vi "Scaling Params.vi"(8 "error in (no error)":errorcluster, 11 "Scaling in":refnum<class "Scaling Config.lvclass">) -> (0 "error out":errorcluster, 1 "Scale Params":dbl[][](array[numeric]), 2 "Scale Types":T1[](array[typedef]), 3 "Scaling out":refnum<class "Scaling Config.lvclass">)   [LabVIEW 2020, in "VolatusConfig.lvlib" / "Scaling Config.lvclass"]
uses:
  Scaling Config.lvclass
  C:/dev/lv20CE/relink/lv-volatus/VolatusConfig/VolatusConfigElement/VolatusConfigElement.lvclass
  Scale Type.ctl
  Meta Type.ctl
  SensorList/SensorList.lvclass
  Scaling Config.lvclass/Scaling Config.ctl
  VolatusConfigElement/VolatusConfigElement.lvclass/VolatusConfigElement.ctl
  VolatusConfigElement/Element.vi
  lv-cdm/CDM-Config/Config Lookup/Match Meta.vi
  lv-cdm/CDM-Config/Config Element/Owner.vi
  lv-cdm/CDM-Config/Config Manager/Lookup Descendant.vi
  lv-cdm/CDM-Config/Config Filter/Config Lookup.lvclass
  VolatusConfigElement/VolatusConfigElement.lvclass
  VolatusConfig.lvlib
  lv-cdm/CDM-Config/Config Element/Config Element.lvclass
  Scale/Scale Config.lvclass
  VolatusErrorUtilities/MultiErrors/MultiErrors.lvclass
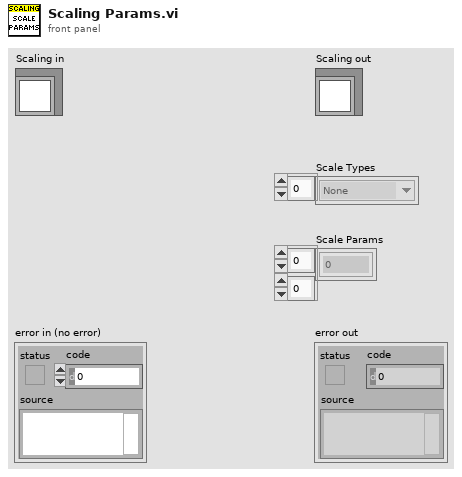
[diagram p1: front panel]
types:
  T1 = typedef "VolatusConfig.lvlib/Scale Type.ctl" = enum16{"None", "Sensor", "Polynomial", "Threshold", "Invert Bool", "Exponential"}
  T2 = typedef "VolatusConfig.lvlib/Meta Type.ctl" = enum16{"UNKNOWN", "VL_System", "VL_Cluster", "VL_Node", "VL_Task", "VL_Group", "VL_Channel", "VL_Task_List", "VL_Scaling", "VL_Sensor", "VL_Sensor_List", "VL_Scale"}
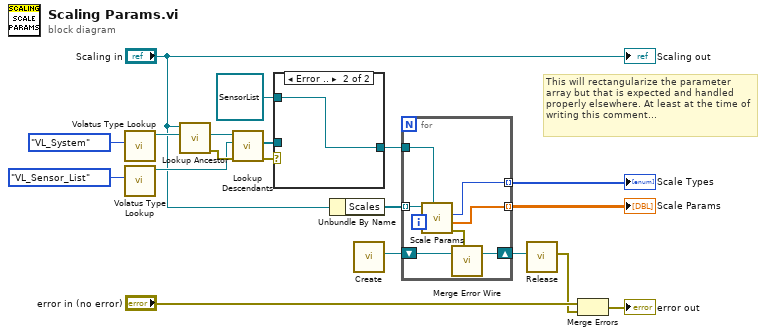
[diagram p0: block diagram]
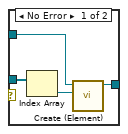
[diagram p2: hidden frame]
diagram:
  # "This will rectangularize the parameter array but that is expected and handled properly elsewhere. At least at the time of writing this comment..."
  n1 = call "Volatus Type Lookup.vi"("Meta Type"=Meta_Type."VL_System") -> ("Config Lookup out"=w18:refnum<class "Config Lookup.lvclass">)  [unwired: 9 in, 1 out]
  n2 = call "Volatus Type Lookup.vi"("Meta Type"=Meta_Type."VL_Sensor_List") -> ("Config Lookup out"=w14:refnum<class "Config Lookup.lvclass">)  [unwired: 9 in, 1 out]
  n3 = call "Lookup Ancestor.vi"("Lookup"=w18, "VolatusConfigElement in"="Scaling in") -> ("error out"=w19:errorcluster, "Ancestor"=w15:refnum<class "Config Element.lvclass">)  [unwired: 7 in, 1 out]
  n4 = call "Lookup Descendants.vi"("error in (no error)"=w19, "Lookup"=w14, "Config Element in"=w15) -> ("error out"=w11:errorcluster, "Descendants"=w13:refnum<class "Config Element.lvclass">[])  [unwired: 6 in, 1 out]
  n5 = case shown="Error .." w11 {
    tunnel: w13 -> [w23 _]
    tunnel: refnum<class "SensorList.lvclass"> refnum ("VolatusConfig.lvlib:SensorList.lvclass") -> [w21 w24]
    tunnel: [w20 w24] -> w9
    frame No Error {
      n6 = Index Array(array=w23) -> (element=w22:refnum<class "Config Element.lvclass">)  [unwired: 1 in]
      n7 = call "Create (Element).vi"("Element"=w22, "VolatusConfigElement in"=w21) -> ("VolatusConfigElement out"=w20:refnum<class "SensorList.lvclass">)  [unwired: 8 in, 1 out]
    }
    frame Error {
    }
  }
  n8 = Unbundle By Name("Scaling in") -> ("Scales"=w8:refnum<class "Scale Config.lvclass">[])
  n9 = call "Create.vi"() -> ("MultiErrors out"=w5:refnum<class "MultiErrors.lvclass">)  [unwired: 11 in]
  n10 = for {
    tunnel: w9 -> [w30]
    tunnel: w8 -> [w31] mode=indexing
    tunnel: [w29] -> w6 mode=indexing
    tunnel: [w28] -> w7 mode=indexing
    shift-right: [w25] -> w4
    shift-left: w5 -> [w27]
    n11 = call "Scale Params.vi"("SensorList (Auto)"=w30, "Scale in"=w31) -> ("error out"=w26:errorcluster, "Scale Params"=w28:dbl[], "Scale Type"=w29:T1)  [unwired: 6 in, 1 out]
    n12 = call "Merge Error Wire.vi"("MultiErrors in"=w27, "error in (no error)"=w26) -> ("MultiErrors out"=w25:refnum<class "MultiErrors.lvclass">)  [unwired: 5 in]
  }
  "Scale Params" <- w7
  "Scale Types" <- w6
  n13 = call "Release.vi"("MultiErrors in"=w4) -> ("error out"=w1:errorcluster)  [unwired: 10 in]
  n14 = Merge Errors("error in (no error)", w1) -> (→"error out":errorcluster)
  "Scaling out" <- "Scaling in"
